vi "Test_init_memory.vi"() -> ()   [LabVIEW 2018]
uses:
  General/Controls/Save Bline to Mem Control.ctl
panel:
  out "error out":errorcluster
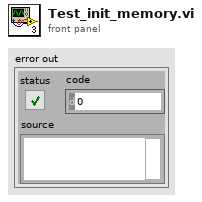
[diagram p1: front panel]
types:
  T1 = typedef "Save Bline to Mem Control.ctl" = enum16{"Output data", "Save(ThorOCT)", "Save(PSOCT)", "FFT and Save", "Uninit", "PSOCT Spectral buffer Set", "PSOCT Spatial buffer Set", "PSOCT Spectral buffer Init", "PSOCT Spatial buffer Init", "ThorOCT Spectral buffer Init", "ThorOCT Spatial buffer Init", "ThorOCT Spectral buffer Set", "ThorOCT Spatial buffer Set", "ThorOCT Spectral Save", "Alazar Spectral Save"}
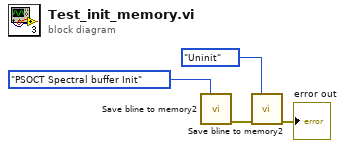
[diagram p0: block diagram]
diagram:
  n1 = call "Save bline to memory2.vi"("action"=Save_Bline_to_Mem_Control."PSOCT Spectral buffer Init") -> ("error out"=w2:errorcluster)  [unwired: 14 in]
  n2 = call "Save bline to memory2.vi"("action"=Save_Bline_to_Mem_Control."Uninit", "error in"=w2) -> ("error out"=→"error out":errorcluster)  [unwired: 13 in]
